vi "AssignDirections.vi"(8 "Actual Angle":dbl, 11 "Target Angle":dbl) -> (0 "Reverse Wheel Direction":bool, 2 "Lowest Angle Error":dbl, 3 "Turn Clockwise":bool)   [LabVIEW 2012, in "ProcessorHelperFunctions.lvlib"]
uses:
  ProcessorHelperFunctions.lvlib
panel:
  out "Error CCW Rev":dbl
  out "Error CW Rev":dbl
  out "Error CCW No Rev":dbl
  out "Error CW No Rev":dbl
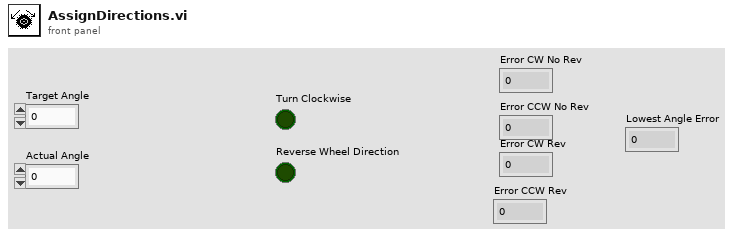
[diagram p1: front panel]
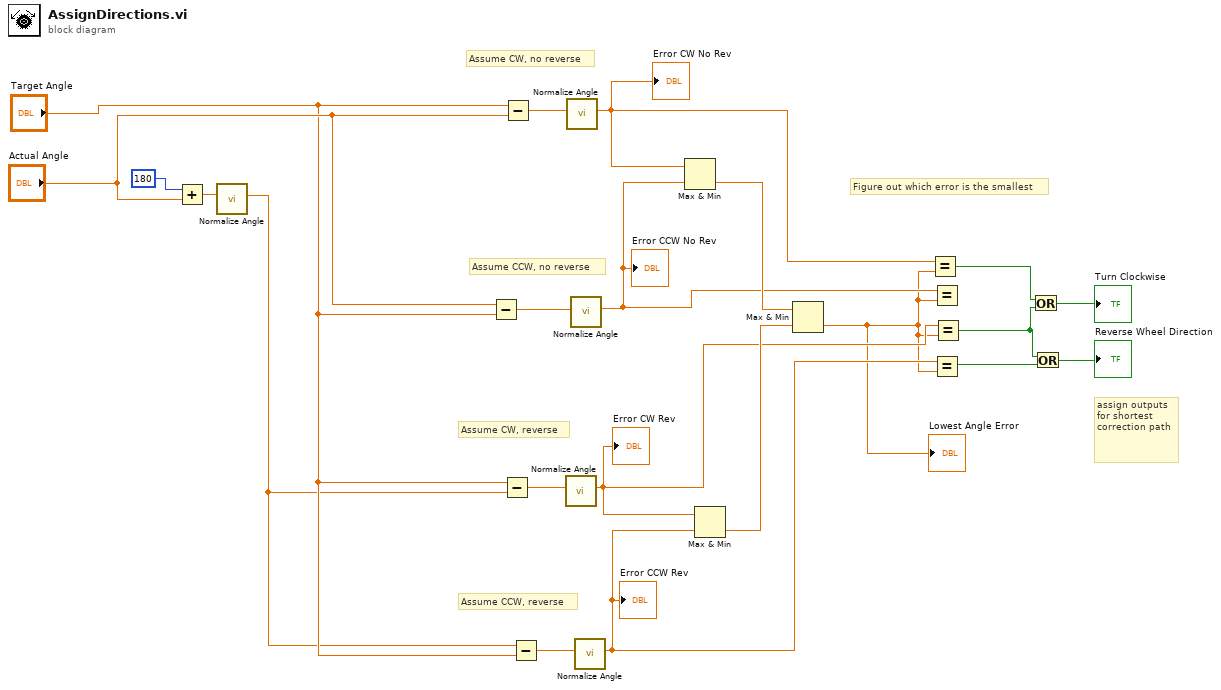
[diagram p0: block diagram]
diagram:
  # "assign outputs for shortest correction path"
  # "Figure out which error is the smallest"
  # "Assume CCW, reverse"
  # "Assume CW, reverse"
  # "Assume CCW, no reverse"
  # "Assume CW, no reverse"
  n1 = Add(x=180, y="Actual Angle") -> (x+y=w17:dbl)
  n2 = call "Normalize Angle.vi"("Input"=w17) -> ("Output"=w13:dbl)  [unwired: 10 in]
  n3 = Subtract(x="Actual Angle", y="Target Angle") -> (x-y=w20:dbl)
  n4 = Subtract(x="Target Angle", y=w13) -> (x-y=w16:dbl)
  n5 = Subtract(x="Target Angle", y="Actual Angle") -> (x-y=w21:dbl)
  n6 = Subtract(x=w13, y="Target Angle") -> (x-y=w15:dbl)
  n7 = call "Normalize Angle.vi"("Input"=w16) -> ("Output"=w8:dbl)  [unwired: 10 in]
  "Error CW Rev" <- w8
  n8 = call "Normalize Angle.vi"("Input"=w21) -> ("Output"=w10:dbl)  [unwired: 10 in]
  "Error CW No Rev" <- w10
  n9 = call "Normalize Angle.vi"("Input"=w20) -> ("Output"=w9:dbl)  [unwired: 10 in]
  "Error CCW No Rev" <- w9
  n10 = call "Normalize Angle.vi"("Input"=w15) -> ("Output"=w7:dbl)  [unwired: 10 in]
  "Error CCW Rev" <- w7
  n11 = Max & Min(x=w10, y=w9) -> (min(x,y)=w12:dbl)  [unwired: 1 out]
  n12 = Max & Min(x=w8, y=w7) -> (min(x,y)=w11:dbl)  [unwired: 1 out]
  n13 = Max & Min(x=w12, y=w11) -> (min(x,y)=w1:dbl)  [unwired: 1 out]
  "Lowest Angle Error" <- w1
  n14 = Equal?(x=w10, y=w1) -> (x = y?=w5:bool)
  n15 = Equal?(x=w9, y=w1) -> ()  [unwired: 1 out]
  n16 = Equal?(x=w7, y=w1) -> (x = y?=w2:bool)
  n17 = Equal?(x=w8, y=w1) -> (x = y?=w3:bool)
  n18 = Or(x=w5, y=w3) -> (x .or. y?=→"Turn Clockwise":bool)
  n19 = Or(x=w3, y=w2) -> (x .or. y?=→"Reverse Wheel Direction":bool)
